vi "sort channels.vi"(8 "error in":errorcluster, 11 "UDP Broadcaster Configuration in":refnum<class "TEC configuration.lvclass">) -> (0 "error out":errorcluster, 3 "UDP Broadcaster Configuration out":refnum<class "TEC configuration.lvclass">)   [LabVIEW 2013, in "TEC configuration.lvclass"]
uses:
  TEC configuration.lvclass
  TEC configuration.lvclass/TEC configuration.ctl
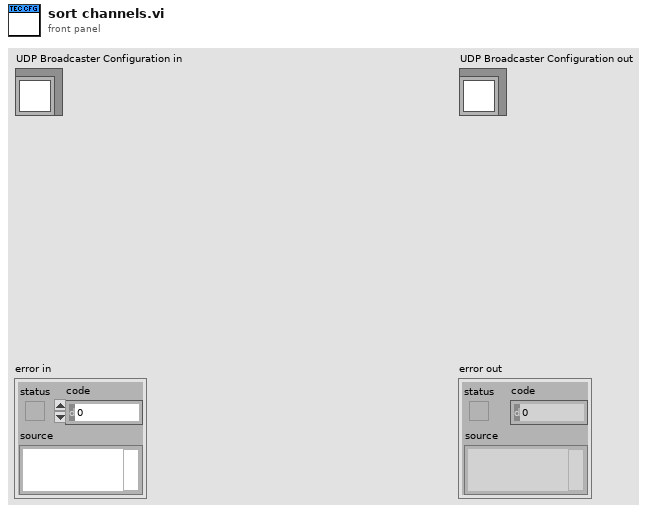
[diagram p1: front panel]
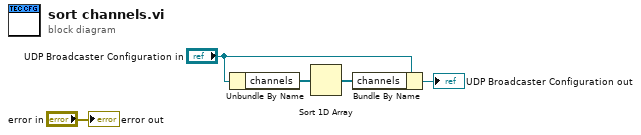
[diagram p0: block diagram]
diagram:
  n1 = Unbundle By Name("UDP Broadcaster Configuration in") -> ("channels"=w2:refnum<class "TBM channel.lvclass">[])
  n2 = Sort 1D Array(array=w2) -> (sorted array=w1:refnum<class "TBM channel.lvclass">[])
  n3 = Bundle By Name(cluster="UDP Broadcaster Configuration in", "channels"=w1) -> (→"UDP Broadcaster Configuration out":refnum<class "TEC configuration.lvclass">)
  "error out" <- "error in"
